vi "EOL Check False Reversal.vi"(11 "AP Data Graph PR GL 3":i16[][](graph)) -> (1 "False Reversal Position":string, 3 "False Reversal?":bool)   [LabVIEW 2018]
panel:
  out "AP Data Graph PR GL 4":i16[](graph)
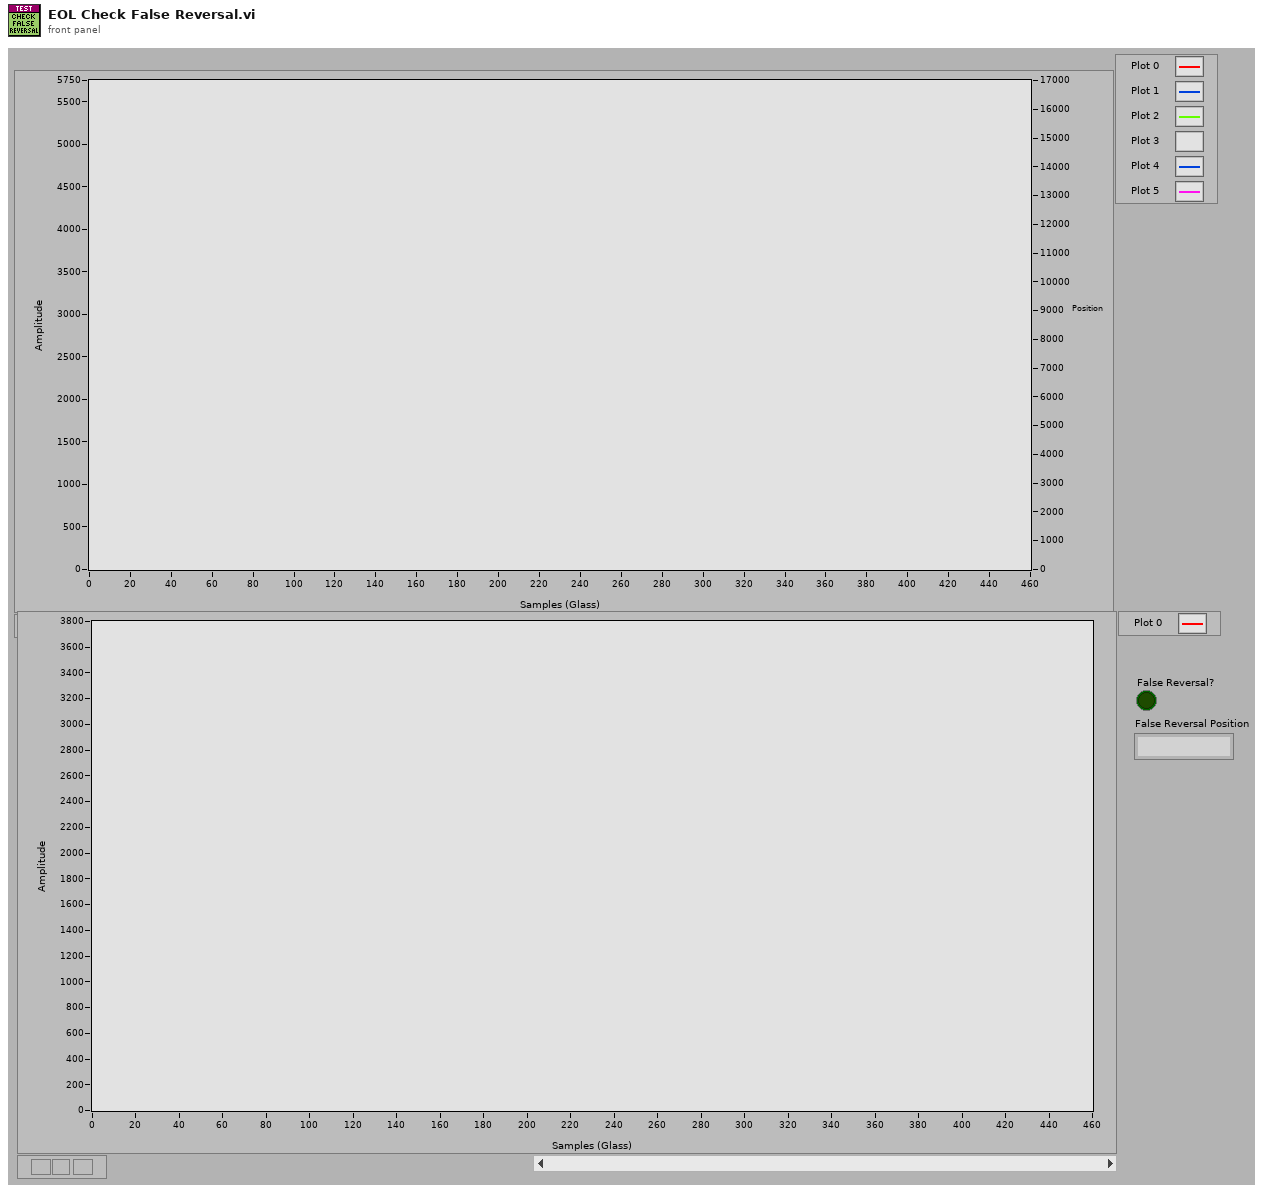
[diagram p1: front panel]
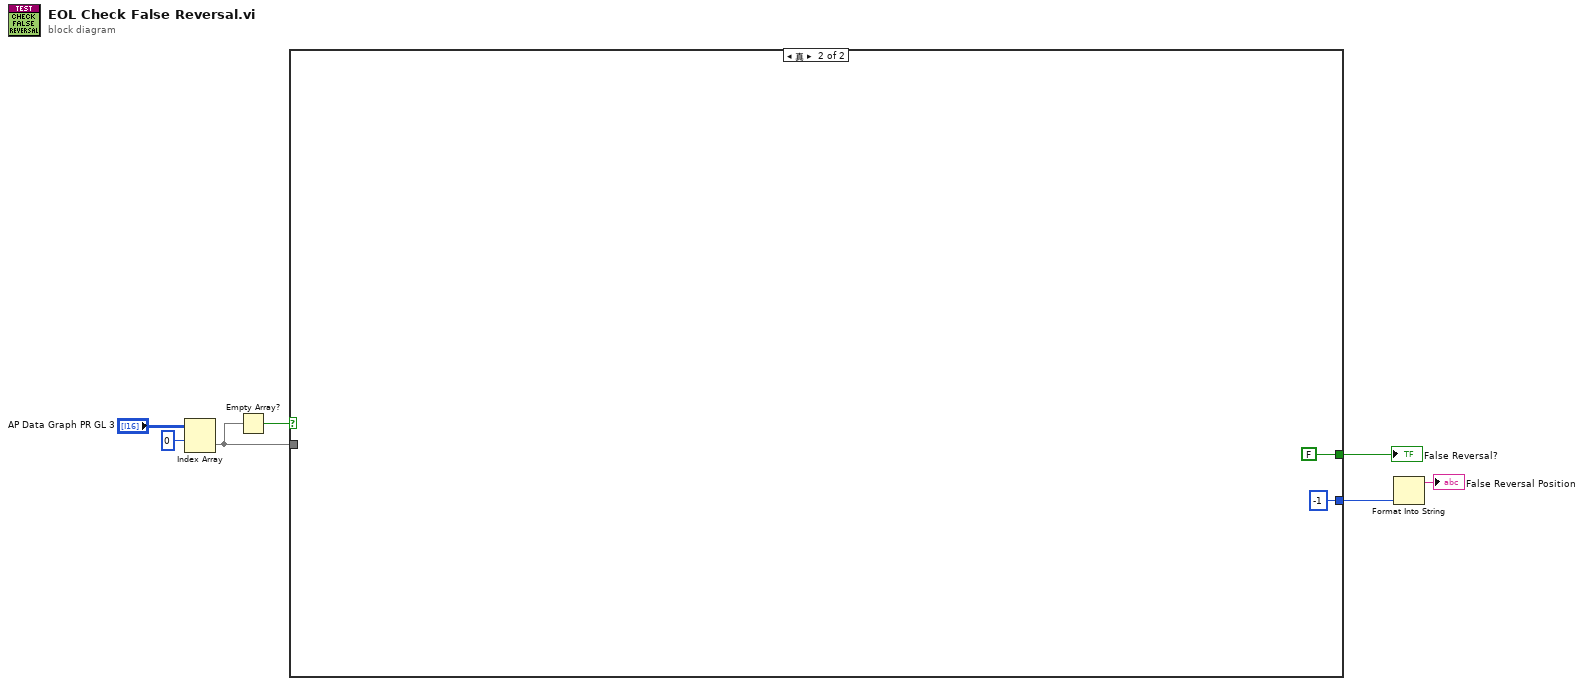
[diagram p0: block diagram]
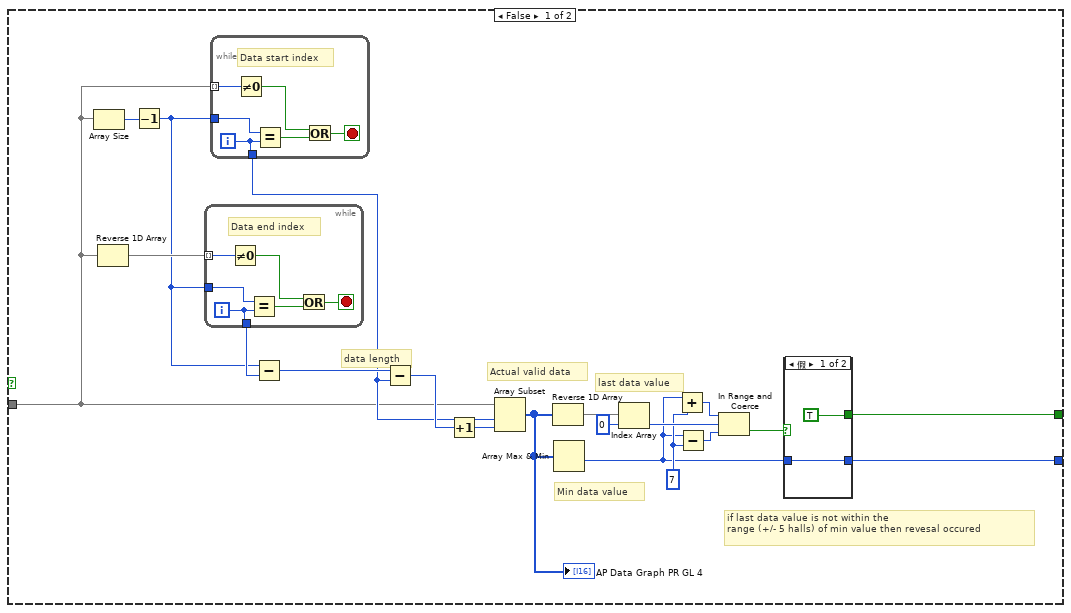
[diagram p2: hidden frame]
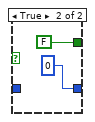
[diagram p3: hidden frame]
diagram:
  n1 = Index Array(array="AP Data Graph PR GL 3", index (row)=0) -> (element=w2:i16[])  [unwired: 1 in]
  n2 = Empty Array?(array=w2) -> (empty?=w1:bool)
  n3 = case shown="真" w1 {
    tunnel: [w11 FALSE] -> w5
    tunnel: [w10 i16 -1 ("f")] -> w4
    tunnel: w2 -> [w8 _]
    frame False {
      w14 = i16 7 ("y")
      # "if last data value is not within the\nrange (+/- 5 halls) of min value then revesal occured"
      # "data length"
      # "Min data value"
      # "last data value"
      # "Actual valid data"
      n4 = Array Size(array=w8) -> (size(s)=w25:i32)
      n5 = Reverse 1D Array(array=w8) -> (reversed array=w24:i16[])
      n6 = Decrement(x=w25) -> (x-1=w19:i32)
      n7 = while {
        tunnel: w24 -> [w37] mode=indexing
        tunnel: w19 -> [w36]
        tunnel: [w32] -> w23
        i -> [w32]
        stop <- w34 stop-if-true
        # "Data end index"
        n8 = Not Equal To 0?(x=w37) -> (x != 0?=w33:bool)
        n9 = Equal?(x=w36, y=w32) -> (x = y?=w35:bool)
        n10 = Or(x=w33, y=w35) -> (x .or. y?=w34:bool)
      }
      n11 = while {
        tunnel: w8 -> [w43] mode=indexing
        tunnel: w19 -> [w42]
        tunnel: [w38] -> w20
        i -> [w38]
        stop <- w40 stop-if-true
        # "Data start index"
        n12 = Not Equal To 0?(x=w43) -> (x != 0?=w39:bool)
        n13 = Equal?(x=w42, y=w38) -> (x = y?=w41:bool)
        n14 = Or(x=w39, y=w41) -> (x .or. y?=w40:bool)
      }
      n15 = Subtract(x=w19, y=w23) -> (x-y=w22:i32)
      n16 = Subtract(x=w22, y=w20) -> (x-y=w21:i32)
      n17 = Increment(x=w21) -> (x+1=w9:i32)
      n18 = Array Subset(array=w8, index=w20, length=w9) -> (w18:i16[])
      "AP Data Graph PR GL 4" <- w18
      n19 = Reverse 1D Array(array=w18) -> (reversed array=w27:i16[])
      n20 = Array Max & Min(array=w18) -> (min value=w12:i16)  [unwired: 3 out]
      n21 = Index Array(array=w27, index=0) -> (element=w17:i16)
      n22 = Add(x=w12, y=w14) -> (x+y=w16:i16)
      n23 = Subtract(x=w12, y=w14) -> (x-y=w15:i16)
      n24 = In Range and Coerce(upper limit=w16, x=w17, lower limit=w15) -> (In Range?=w13:bool)  [unwired: 1 out]
      n25 = case shown="假" w13 {
        tunnel: w12 -> [w29 _]
        tunnel: [w29 i16 0 ("f")] -> w10
        tunnel: [TRUE FALSE] -> w11
        frame False {
        }
        frame True {
        }
      }
    }
    frame True {
    }
  }
  "False Reversal?" <- w5
  n26 = Format Into String(w4) -> (resulting string=→"False Reversal Position":string)  [unwired: 3 in, 1 out]
